vi "MQTT_10Hz.vi"(7 "string":string="Raw.DMG_MORI_DMU_40_EVO", 9 "data 2":dbl[](array[numeric]), 10 "Machine Data":T1={"Zload"="", "Yload"="", "Xload"="", "path_position"="", "Fovr"="", "SspeedOvr"="", "Program Name"="", "Program status"="", "Block of code being executed"="", "Line of code"="", "Machine availability"="", "Emergency status"="", "Controller mode"="", "Tool_id"="UNAVAILABLE"}, 11 "current time 2":timestamp) -> (3 "JSON string":string)   [LabVIEW 2017]
uses:
  UI Error Handlers/support/data_base_structure.ctl
panel:
  out "current time 3":timestamp
  out "resulting string 2":string
  out "Xload":string
  out "Machine availability":string
  out "resulting string":string
  out "output array 2":dbl[](array[numeric])
  out "size(s) 2":i32
  out "valueSent 2":string="14:19:17.238_"
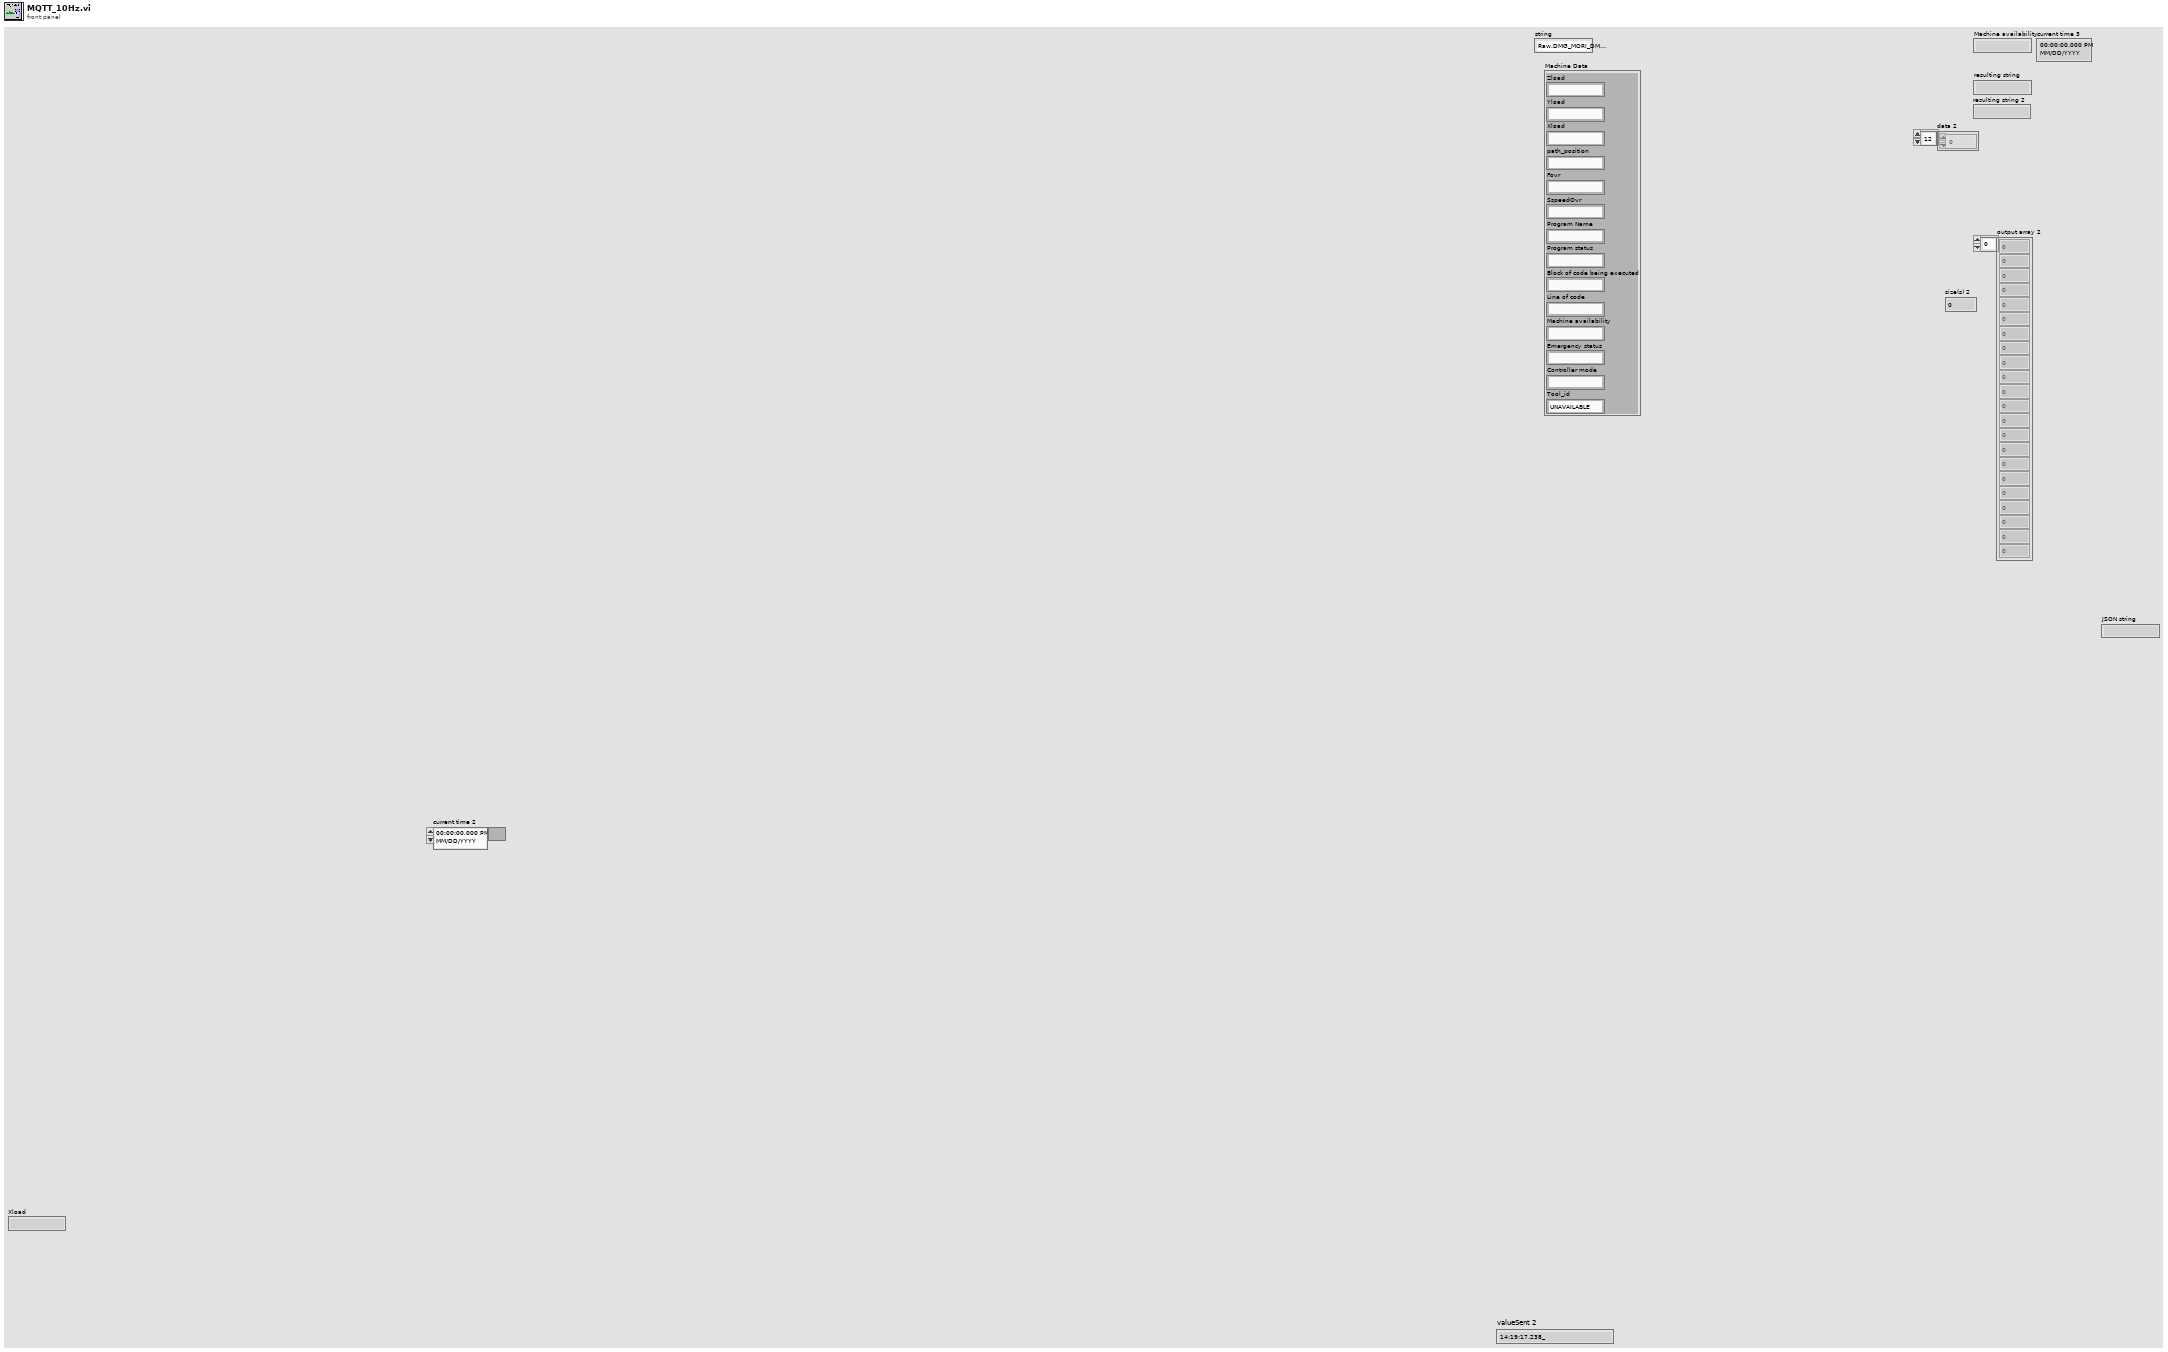
[diagram p1: front panel]
types:
  T1 = cluster{"Zload":string, "Yload":string, "Xload":string, "path_position":string, "Fovr":string, "SspeedOvr":string, "Program Name":string, "Program status":string, "Block of code being executed":string, "Line of code":string, "Machine availability":string, "Emergency status":string, "Controller mode":string, "Tool_id":string}
  T2 = enum8{"Enabled", "Disabled", "Disabled and Grayed Out"}
  T3 = typedef "data_base_structure.ctl" = cluster{"available ":dbl, "controller_mode":string, "spindle_load":dbl, "spindle_speed ":dbl, "sspeedovr":dbl, "J_part":dbl, "K_part":dbl, "Xpos_part":dbl, "Ypos_part":dbl, "Zpos_part":dbl, "Apos_machine":dbl, "Bpos_machine":dbl, "Xload":dbl, "Yload":dbl, "Zload":dbl, "Aload":dbl, "Bload":dbl, "tool_id":dbl, "program_name":string, "block_code":string, "line_number":dbl, "estop":string, "accel_x_rms":dbl, "accel_y_rms":dbl, "accel_z_rms":dbl, "program_number":dbl, "timestamp":string, "feed_rate ":dbl, "fovr":dbl, "I_part ":dbl}
  T4 = cluster{"date/time string":string, "available":string, "Controller mode":string, "spindle_load":dbl, "spindle_speed":dbl, "sspeedovr":dbl, "feed_rate":dbl, "fovr":dbl, "I_part":dbl, "J_part":dbl, "K_part":dbl, "Xpos_part":dbl, "Ypos_part":dbl, "Zpos_part":dbl, "Apos_machine":dbl, "Bpos_machine":dbl, "Xload":dbl, "Yload":dbl, "Zload":dbl, "Aload":dbl, "Bload":dbl, "tool_id":dbl, "program_number":dbl, "Program Name":string, "Block of code being executed":string, "line_number":dbl, "Emergency status":string, "accel_x_rms":dbl, "accel_y_rms":dbl, "accel_z_rms":dbl}
  T5 = cluster{"date/time string":string, "Machine availability":string}
  T6 = cluster{"data 2[0]":dbl, "data 2[1]":dbl, "data 2[2]":dbl, "data 2[3]":dbl, "data 2[4]":dbl, "data 2[5]":dbl, "data 2[6]":dbl, "data 2[7]":dbl, "data 2[8]":dbl, "data 2[9]":dbl, "data 2[10]":dbl, "data 2[11]":dbl, "data 2[12]":dbl, "data 2[13]":dbl, "data 2[14]":dbl, "data 2[15]":dbl, "data 2[16]":dbl, "data 2[17]":dbl, "data 2[18]":dbl, "data 2[19]":dbl, "data 2[20]":dbl, "data 2[21]":dbl}
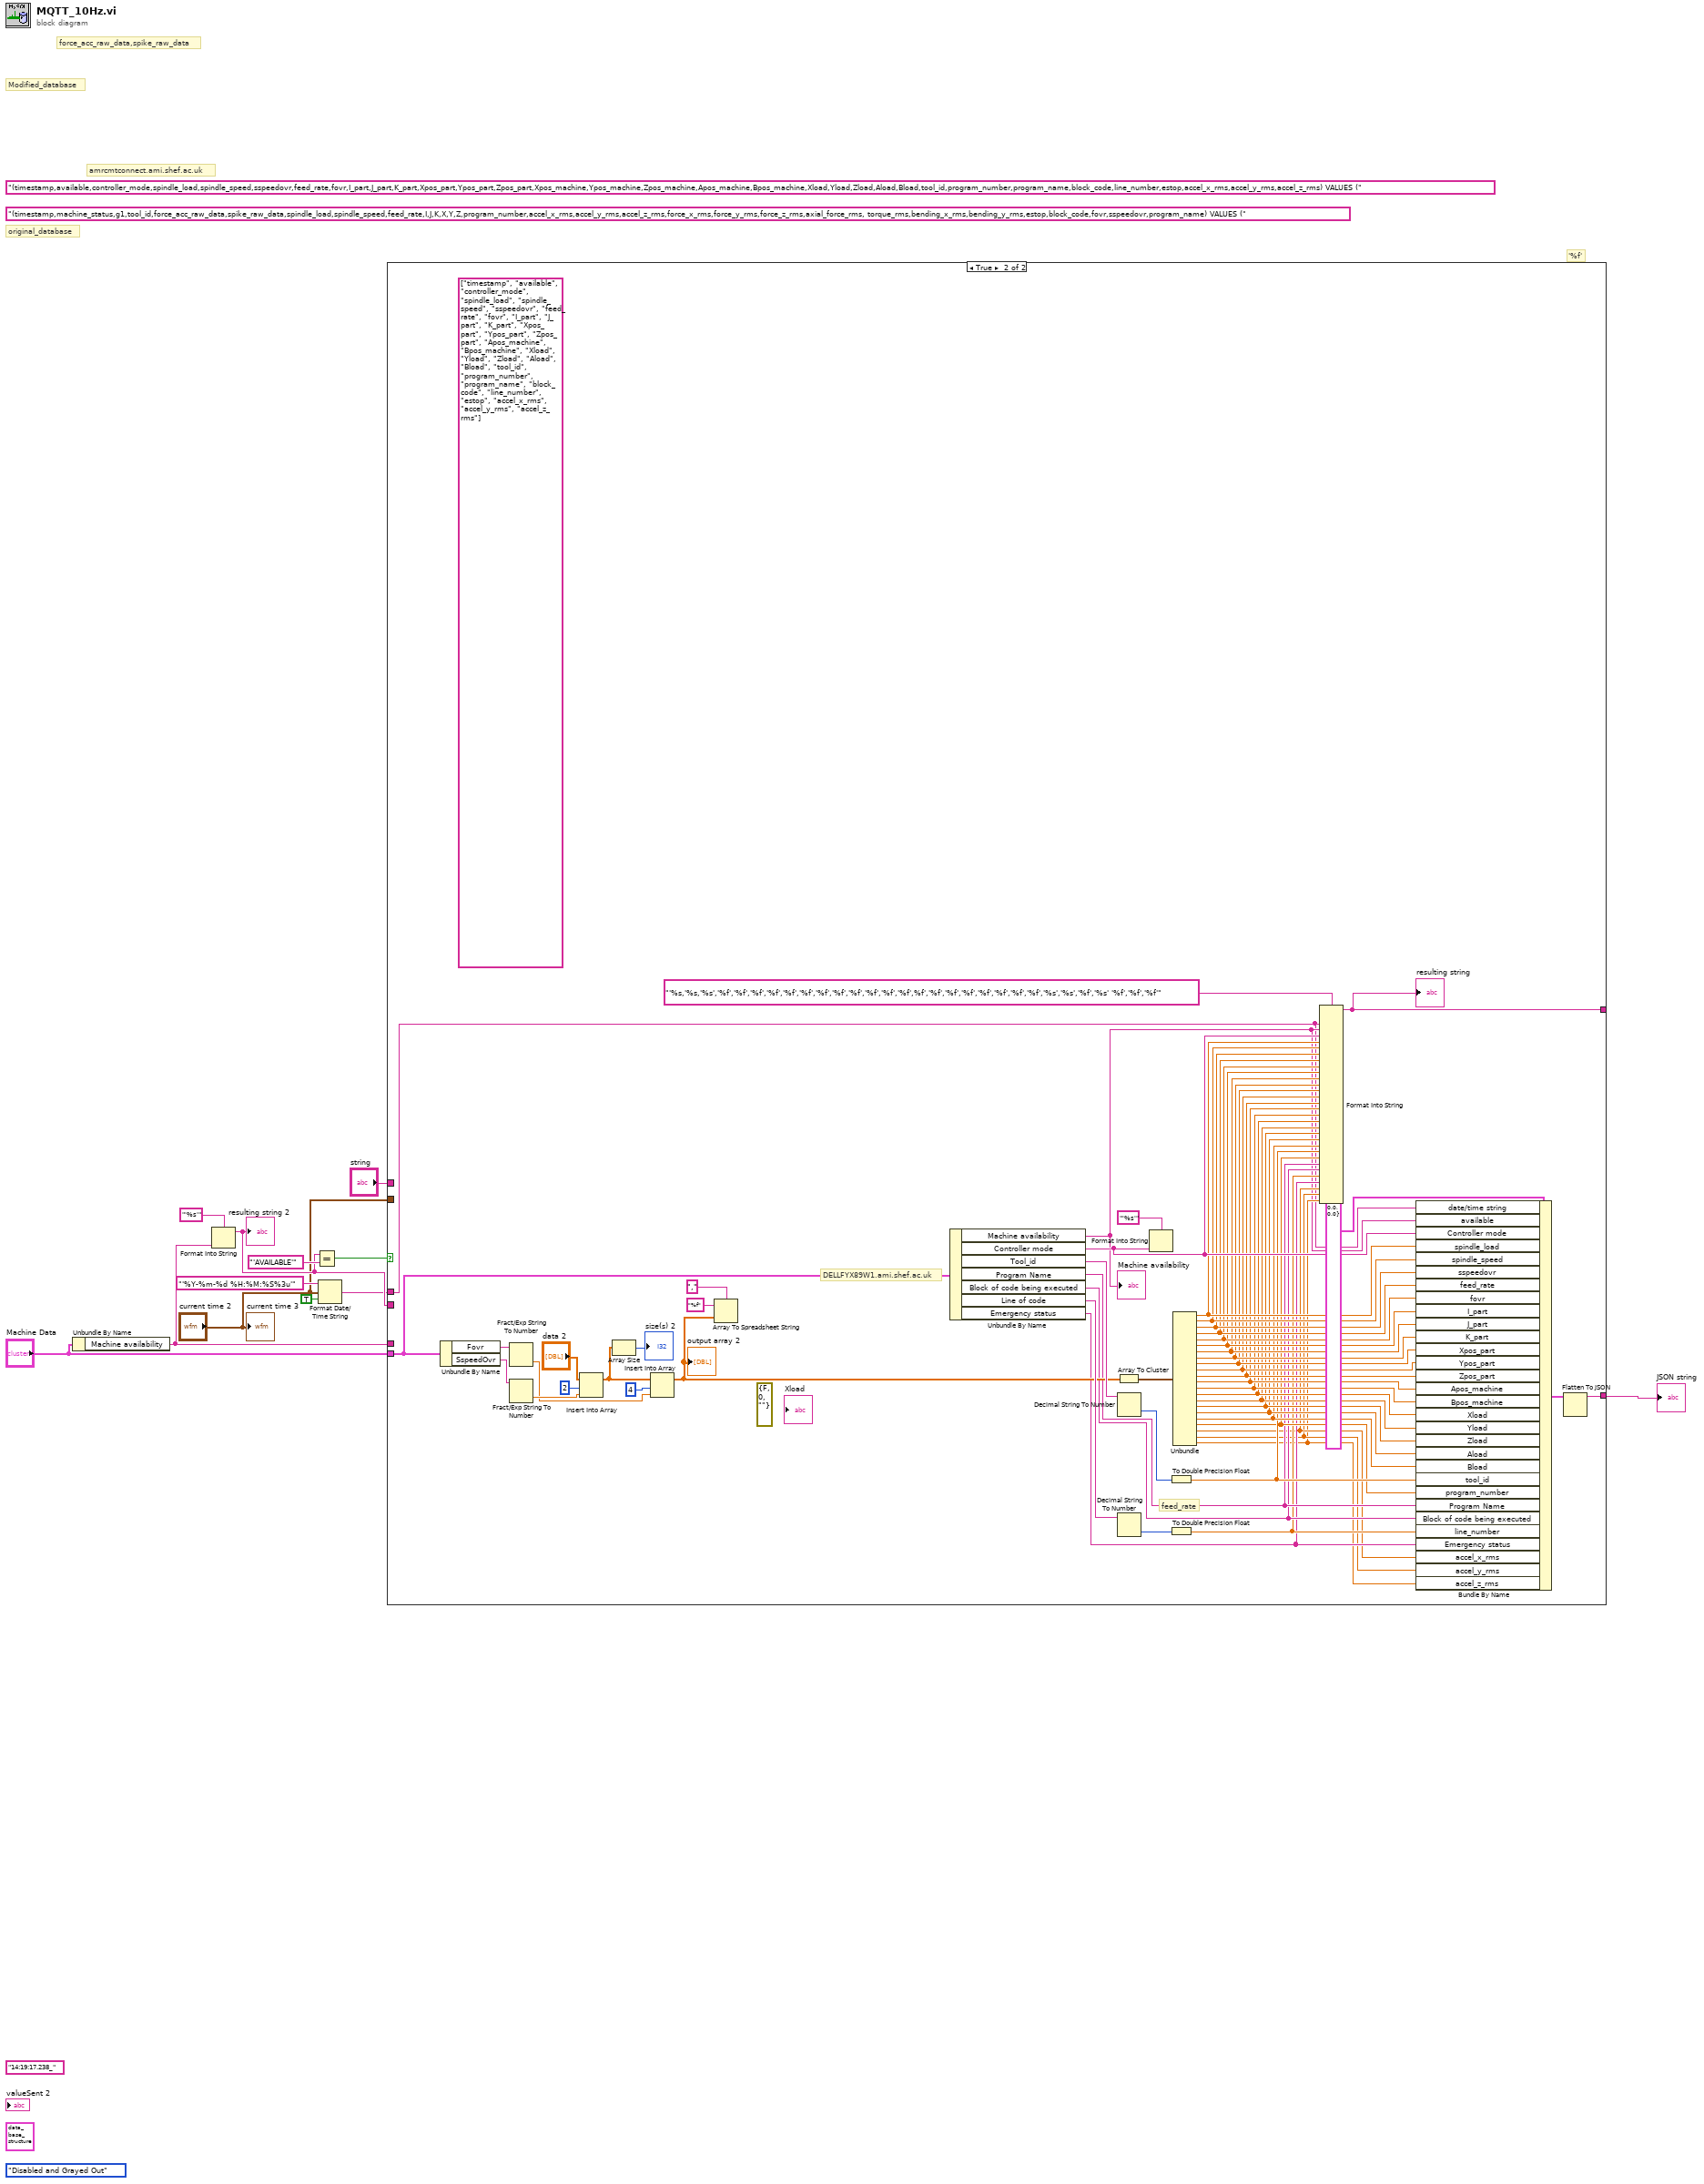
[diagram p0: block diagram]
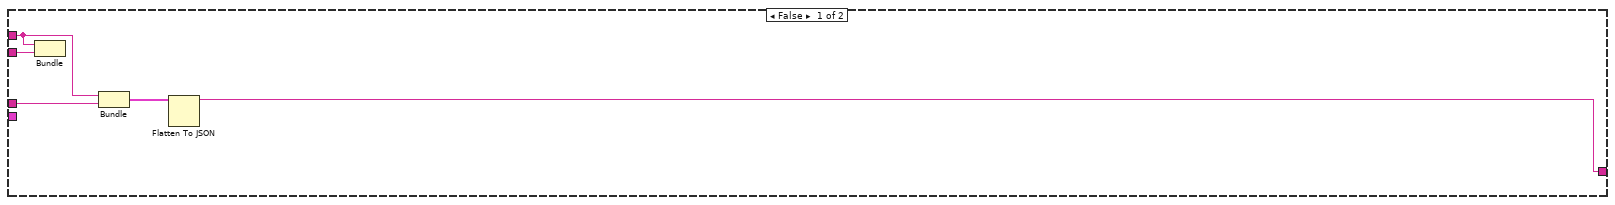
[diagram p2: hidden frame]
diagram:
  (unwired) T2."Disabled and Grayed Out" ("Disabled")
  (unwired) "14:19:17.238_" ("valueSent 2")
  (unwired) T3 {"available "=0.0, "controller_mode"="", "spindle_load"=0.0, "spindle_speed "=0.0, "sspeedovr"=0.0, "J_part"=0.0, "K_part"=0.0, "Xpos_part"=0.0, "Ypos_part"=0.0, "Zpos_part"=0.0, "Apos_machine"=0.0, "Bpos_machine"=0.0, "Xload"=0.0, "Yload"=0.0, "Zload"=0.0, "Aload"=0.0, "Bload"=0.0, "tool_id"=0.0, "program_name"="", "block_code"="", "line_number"=0.0, "estop"="", "accel_x_rms"=0.0, "accel_y_rms"=0.0, "accel_z_rms"=0.0, "program_number"=0.0, "timestamp"="", "feed_rate "=0.0, "fovr"=0.0, "I_part "=0.0} ("Cluster")
  (unwired) "(timestamp,available,controller_mode,spindle_load,spindle_speed,sspeedovr,feed_rate,fovr,I_part,J_part,K_part,Xpos_part,Ypos_part,Zpos_part,Xpos_machine,Ypos_machine,Zpos_machine,Apos_machine,Bpos_machine,Xload,Yload,Zload,Aload,Bload,tool_id,program_number,program_name,block_code,line_number,estop,accel_x_rms,accel_y_rms,accel_z_rms) VALUES (" ("string")
  (unwired) "(timestamp,machine_status,g1,tool_id,force_acc_raw_data,spike_raw_data,spindle_load,spindle_speed,feed_rate,I,J,K,X,Y,Z,program_number,accel_x_rms,accel_y_rms,accel_z_rms,force_x_rms,force_y_rms,force_z_rms,axial_force_rms, torque_rms,bending_x_rms,bending_y_rms,estop,block_code,fovr,sspeedovr,program_name) VALUES (" ("string")
  # "'%f'"
  # "original_database"
  # "force_acc_raw_data,spike_raw_data"
  # "Modified_database"
  # "amrcmtconnect.ami.shef.ac.uk"
  n1 = Unbundle By Name("Machine Data") -> ("Machine availability"=w3:string)
  n2 = Format Into String(format string="'%s'", w3) -> (resulting string=w6:string)  [unwired: 2 in, 1 out]
  "resulting string 2" <- w6
  n3 = Equal?(x=w6, y="'AVAILABLE'") -> (x = y?=w8:bool)
  n4 = Format Date/Time String(time format string (%c)="'%Y-%m-%d %H:%M:%S%3u'", seconds (now)="current time 2", UTC format=TRUE) -> (date/time string=w4:string)
  n5 = case shown="True" w8 {
    tunnel: [_ w21] -> _
    tunnel: "Machine Data" -> [_ w23]
    tunnel: "string" -> [_ _]
    tunnel: w6 -> [w17 _]
    tunnel: "current time 2" -> [_ _]
    tunnel: w4 -> [w15 w20]
    tunnel: [w13 w18] -> w2
    tunnel: w3 -> [w16 _]
    frame False {
      n6 = Bundle("date/time string"=w15, w17) -> ()  [unwired: 1 in, 1 out]
      n7 = Bundle("date/time string"=w15, "Machine availability"=w16) -> (w14:T5)  [unwired: 1 in]
      n8 = Flatten To JSON(anything=w14) -> (JSON string=w13:string)  [unwired: 2 in, 1 out]
    }
    frame True {
      (unwired) errorcluster {"status"=FALSE, "code"=0, "source"=""} ("error out")
      (unwired) string[] ["timestamp", "available", "controller_mode", "spindle_load", "spindle_speed", "sspeedovr", "feed_rate", "fovr", "I_part", "J_part", "K_part", "Xpos_part", "Ypos_part", "Zpos_part", "Apos_machine", "Bpos_machine", "Xload", "Yload", "Zload", "Aload", "Bload", "tool_id", "program_number", "program_name", "block_code", "line_number", "estop", "accel_x_rms", "accel_y_rms", "accel_z_rms"]
      # "feed_rate"
      # "DELLFYX89W1.ami.shef.ac.uk"
      n9 = Unbundle By Name(w23) -> ("Fovr"=w63:string, "SspeedOvr"=w68:string)
      n10 = Fract/Exp String To Number(string=w63) -> (number=w65:dbl)  [unwired: 3 in, 1 out]
      n11 = Fract/Exp String To Number(string=w68) -> (number=w67:dbl)  [unwired: 3 in, 1 out]
      n12 = Insert Into Array(array="data 2", index=2, new element=w67) -> (w61:dbl[])
      n13 = Array Size(array=w61) -> (size(s)=→"size(s) 2":i32)
      n14 = Insert Into Array(array=w61, index=4, new element=w65) -> (w55:dbl[])
      "output array 2" <- w55
      n15 = Array To Spreadsheet String(delimiter (Tab)=",", array=w55, 3:"%f" ("format string")) -> ()  [unwired: 1 out]
      n16 = Unbundle By Name(w23) -> ("Machine availability"=w24:string, "Controller mode"=w52:string, "Tool_id"=w59:string, "Program Name"=w31:string, "Block of code being executed"=w30:string, "Line of code"=w58:string, "Emergency status"=w28:string)
      "Machine availability" <- w24
      n17 = Array To Cluster(array=w55) -> (cluster=w54:T6)
      n18 = Decimal String To Number(string=w59) -> (number=w60:i32)  [unwired: 2 in, 1 out]
      n19 = Decimal String To Number(string=w58) -> (number=w57:i32)  [unwired: 2 in, 1 out]
      n20 = Format Into String(format string="'%s'", w52) -> ()  [unwired: 2 in, 2 out]
      n21 = To Double Precision Float(number=w60) -> (double precision float=w33:dbl)
      n22 = To Double Precision Float(number=w57) -> (double precision float=w29:dbl)
      n23 = Unbundle(w54) -> ("data 2[0]"=w51:dbl, "data 2[1]"=w50:dbl, "data 2[2]"=w49:dbl, "data 2[3]"=w48:dbl, "data 2[4]"=w47:dbl, "data 2[5]"=w46:dbl, "data 2[6]"=w45:dbl, "data 2[7]"=w44:dbl, "data 2[8]"=w43:dbl, "data 2[9]"=w42:dbl, "data 2[10]"=w41:dbl, "data 2[11]"=w40:dbl, "data 2[12]"=w39:dbl, "data 2[13]"=w38:dbl, "data 2[14]"=w37:dbl, "data 2[15]"=w36:dbl, "data 2[16]"=w35:dbl, "data 2[17]"=w34:dbl, "data 2[18]"=w32:dbl, "data 2[19]"=w27:dbl, "data 2[20]"=w26:dbl, "data 2[21]"=w25:dbl)
      n24 = Format Into String(format string="'%s,'%s,'%s','%f','%f','%f','%f','%f','%f','%f','%f','%f','%f','%f','%f',%f','%f','%f','%f','%f','%f','%f','%f','%s','%s','%f','%s' '%f','%f','%f'", w20, w24, w52, w51, w50, w49, w48, w47, w46, w45, w44, w43, w42, w41, w40, w39, w38, w37, w36, w35, w34, w33, w32, w31, w30, w29, w28, w27, w26, w25) -> (resulting string=w21:string)  [unwired: 2 in, 1 out]
      "resulting string" <- w21
      n25 = Bundle By Name(cluster=T4 {"date/time string"="", "available"="", "Controller mode"="", "spindle_load"=0.0, "spindle_speed"=0.0, "sspeedovr"=0.0, "feed_rate"=0.0, "fovr"=0.0, "I_part"=0.0, "J_part"=0.0, "K_part"=0.0, "Xpos_part"=0.0, "Ypos_part"=0.0, "Zpos_part"=0.0, "Apos_machine"=0.0, "Bpos_machine"=0.0, "Xload"=0.0, "Yload"=0.0, "Zload"=0.0, "Aload"=0.0, "Bload"=0.0, "tool_id"=0.0, "program_number"=0.0, "Program Name"="", "Block of code being executed"="", "line_number"=0.0, "Emergency status"="", "accel_x_rms"=0.0, "accel_y_rms"=0.0, "accel_z_rms"=0.0}, "date/time string"=w20, "available"=w24, "Controller mode"=w52, "spindle_load"=w51, "spindle_speed"=w50, "sspeedovr"=w49, "feed_rate"=w48, "fovr"=w47, "I_part"=w46, "J_part"=w45, "K_part"=w44, "Xpos_part"=w43, "Ypos_part"=w42, "Zpos_part"=w41, "Apos_machine"=w40, "Bpos_machine"=w39, "Xload"=w38, "Yload"=w37, "Zload"=w36, "Aload"=w35, "Bload"=w34, "tool_id"=w33, "program_number"=w32, "Program Name"=w31, "Block of code being executed"=w30, "line_number"=w29, "Emergency status"=w28, "accel_x_rms"=w27, "accel_y_rms"=w26, "accel_z_rms"=w25) -> (w19:T4)
      n26 = Flatten To JSON(anything=w19) -> (JSON string=w18:string)  [unwired: 2 in, 1 out]
    }
  }
  "JSON string" <- w2
  "current time 3" <- "current time 2"
